vi "Periodic Tasks.vi"(8 "error in":errorcluster) -> ()   [LabVIEW 2016]
doc: "This VI runs in parallel to other tasks. It can contain as many user-defined periodic loops as you need. These can carry out PID or other sorts of timed response."
uses:
  Control 1.ctl
  <vilib>/Platform/TimedLoop/XDataNode/timing_clust.ctl
  <vilib>/Platform/TimedLoop/XDataNode/nitl_modes.ctl
  <vilib>/Platform/TimedLoop/XDataNode/wakeup.ctl
  <userlib>/836-Library/Drive/Drive_Code_V2/Drive_Code_Support/SensorTypedefs/Sensor_Cluster.ctl
  <userlib>/836-Library/Drive/Drive_Code_V2/Drive_Code_Support/SensorTypedefs/Camera_Cluster.ctl
  <vilib>/Rock Robotics/WPI/RobotDrive/WPI_RobotDriveDevRef.ctl
  <vilib>/Rock Robotics/WPI/MotorControl/WPI_MotorControlDeviceRef.ctl
  <vilib>/Rock Robotics/WPI/MotorControl/WPI_MotorControlType.ctl
  <vilib>/Rock Robotics/SystemInterfaces/DIO/FPGA_DIOPWMChannel.ctl
  <vilib>/Rock Robotics/WPI/PWM/WPI_PWMDeadband.ctl
  <userlib>/836-Library/Drive/Drive_Code_V2/Drive_Code_Support/DriveTrains/Drive_Trains.ctl
  <userlib>/836-Library/Drive/Drive_Code_V2/Drive_Code_Support/Command_Sends/Drive_Code_Command_Type.ctl
  <userlib>/836-Library/Drive/Drive_Code_V2/Drive_Code_Support/Command_Sends/Drive_Code_Command_List.ctl
  <userlib>/836-Library/Drive/Drive_Code_V2/Drive_Code_Support/PidClusters/PidInversions.ctl
  <userlib>/836-Library/Drive/Drive_Code_V2/Drive_Code_Support/PidClusters/DrivePidInputs.ctl
  <userlib>/836-Library/Drive/Drive_Code_V2/Drive_Code_Support/PidClusters/PidInputs.ctl
  <userlib>/836-Library/Drive/Drive_Code_V2/Drive_Code_Support/Command_Sends/Command_Tolerances.ctl
  <userlib>/836-Library/Drive/Drive_Code_V2/Drive_Code_Support/Command_Sends/Command_Tolerance_Info.ctl
  <vilib>/Rock Robotics/WPI/Utilities/WPI_GetSetVariantRefNum.vi
  <userlib>/836-Library/Drive/Drive_Code_V2/Drive_Code_Support/Command_Sends/Drive_Cmd_Cheesey_Drive.vi
  <vilib>/platform/TimedLoop/XDataNode/XDataNode.xnode
  <vilib>/Platform/TimedLoop/XDataNode/XDNodeRunTimeDep.lvlib
panel:
  in  "Tab Control":T1(tab)=enum."Motor_9"
  in  "Press and Hold? 4":T2=TRUE
  in  "Reverse Direction? 4":bool
  in  "Power 4":dbl(knob) scale=0.0..1.0
  in  "Press and Hold? 5":T2=TRUE
  in  "Reverse Direction? 5":bool
  in  "Power 5":dbl(knob) scale=0.0..1.0
  in  "Press and Hold? 6":T2=TRUE
  in  "Reverse Direction? 6":bool
  in  "Power 6":dbl(knob) scale=0.0..1.0
  in  "Press and Hold? 7":T2=TRUE
  in  "Reverse Direction? 7":bool
  in  "Power 7":dbl(knob) scale=0.0..1.0
  in  "Rev Press and Hold? 8":T2=TRUE
  in  "Rev Power 8":dbl(knob) scale=0.0..1.0
  in  "Fwd Press and Hold? 8":T2=TRUE
  in  "Reverse Direction? 8":bool
  in  "Fwd Power 8":dbl(knob) scale=0.0..1.0
  in  "Rev Press and Hold? 9":T2=TRUE
  in  "Rev Power 9":dbl(knob) scale=0.0..1.0
  in  "Fwd Press and Hold? 9":T2=TRUE
  in  "Reverse Direction? 9":bool
  in  "Fwd Power 9":dbl(knob) scale=0.0..1.0
  # "PWM: 4\nButton: X"
  # "PWM: 5\nButton: A"
  # "PWM: 6\nButton: B"
  # "PWM: 7\nButton: Y"
  # "PWM: 8\nFwd Button: RB\nRev Button: LB"
  # "PWM: 9\nFwd Button: RT\nRev Button: LT"
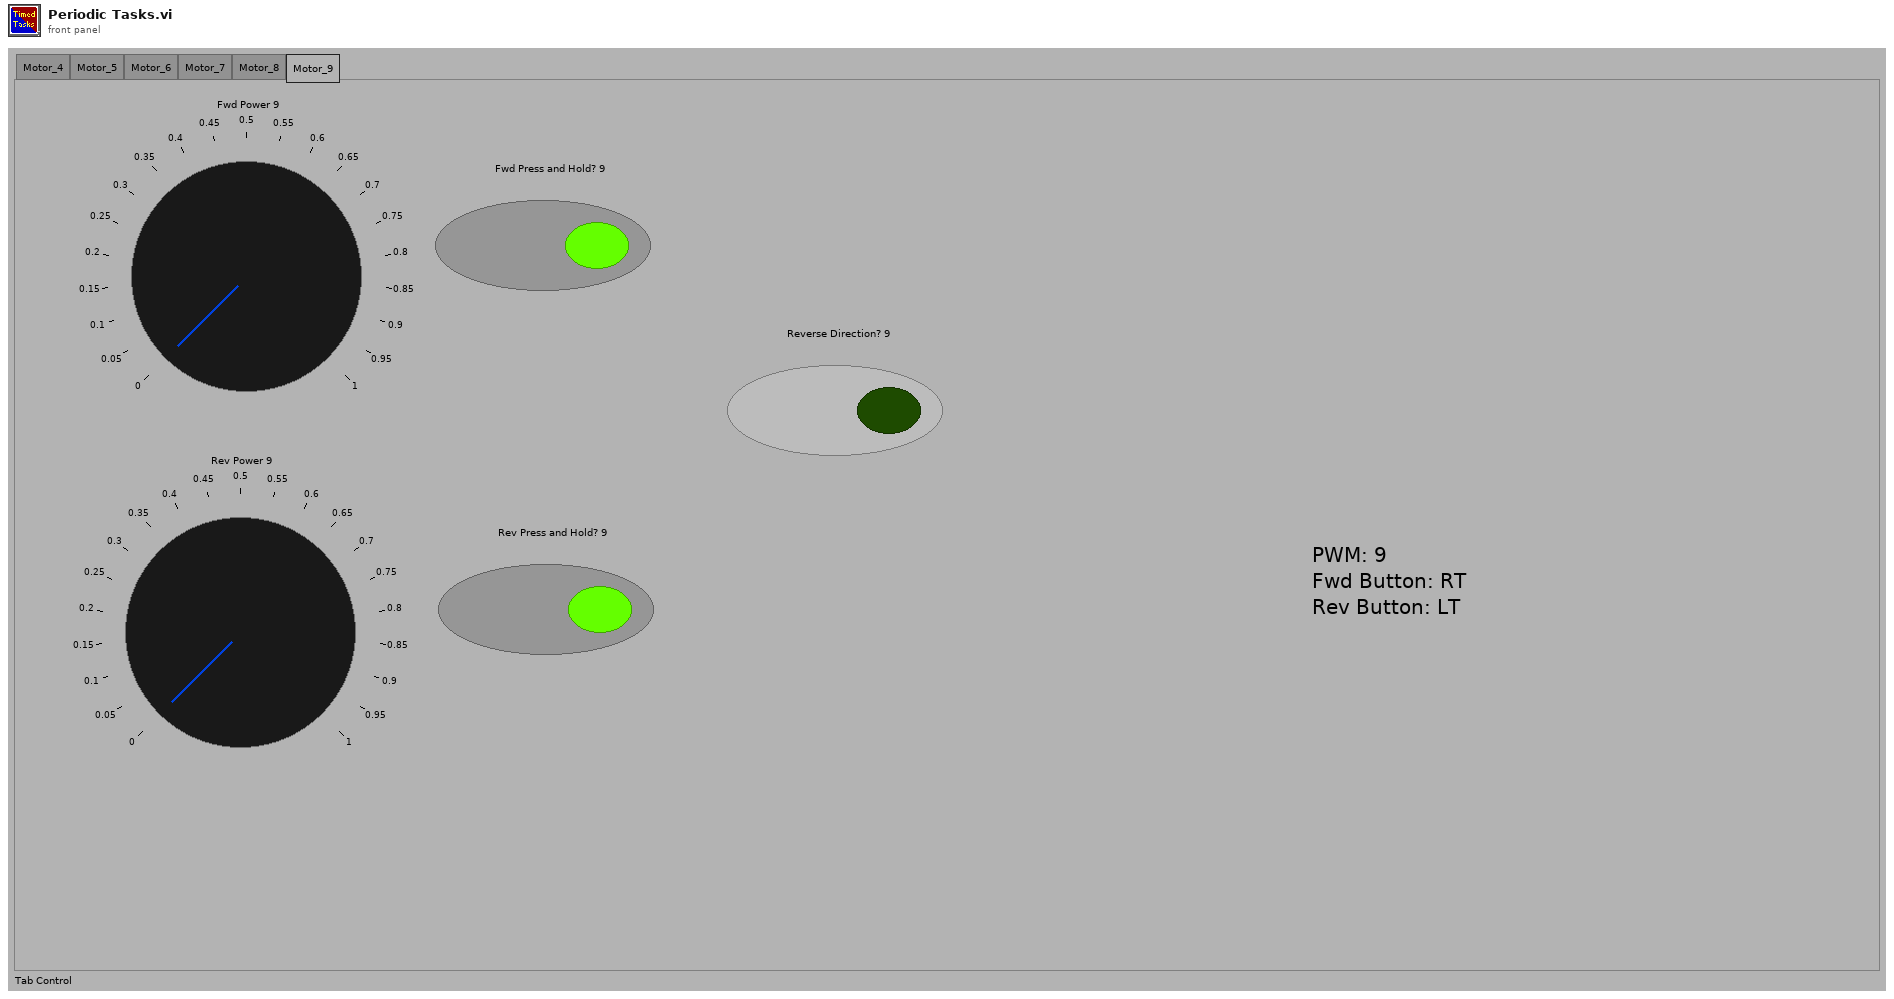
[diagram p1: front panel]
types:
  T1 = enum32{"Motor_4", "Motor_5", "Motor_6", "Motor_7", "Motor_8", "Motor_9"}
  T2 = typedef "Control 1.ctl" = bool
  T3 = typedef "XDNodeRunTimeDep.lvlib/timing_clust.ctl" = cluster{"Expected End [f-1]":u64, "Actual End [f-1]":u64, "Finished Late? [f-1]":bool, "Expected End [i-1]":u64, "Actual End [i-1]":u64, "Finished Late? [i-1]":bool, "Expected Start [i]":u64, "Actual Start [i]":u64, "Expected Start [f]":u64, "Actual Start [f]":u64, "Source Name":string, "Structure Name":string, "Period":i64, "Deadline":i64, "Offset":i64, "Start":i64, "Priority":i32, "Timeout":i32, "Mode":T4, "Wakeup Reason":T5, "Error":errorcluster, "Source Type":string, "Secondary Source Type":string, "Global End Time":u64, "Global Start Time":u64, "Frame Duration":u64, "Iteration Duration":u64, "Assigned CPU":i32, "I/O Scan Engine Mode":u32}
  T4 = typedef "XDNodeRunTimeDep.lvlib/nitl_modes.ctl" = enum32{"No Change", "Process missed periods, maintain original phase", "Discard missed periods, maintain original phase", "Process missed periods, ignore original phase", "Discard missed periods, ignore original phase"}
  T5 = typedef "XDNodeRunTimeDep.lvlib/wakeup.ctl" = enum32{"Normal", "Aborted", "Asynchronous wakeup", "Timing source error", "Timed loop error", "Timeout"}
  T6 = cluster{"Rev Power":dbl, "Rev Press and Hold?":T2}
  T7 = cluster{"Fwd Power":dbl, "Fwd Press and Hold?":T2}
  T8 = typedef "WPI_JoystickDevRef.ctl" = cluster{"Device":T9}
  T9 = typedef "WPI_JoystickDeviceEnum.ctl" = enum16{"USB 0", "USB 1", "USB 2", "USB 3", "USB 4", "USB 5"}
  T10 = typedef "Sensor_Cluster.ctl" = cluster{"Gyro Data":cluster{"Gyro RT FIFO":refnum<k33>, "Gyro Current":dbl, "Gyro Hold":dbl}, "Encoder Data":cluster{"Encoder RT FIFO":refnum<k33>, "Encoder Current":dbl, "Encoder Hold":dbl}, "Camera Data":cluster{"Camera RT FIFO":refnum<k33>, "Camera Current":T11}}
  T11 = typedef "Camera_Cluster.ctl" = cluster{" Angle":dbl, "Valid":bool}
  T12 = typedef "WPI_RobotDriveDevRef.ctl" = cluster{"DevStatus":errorcluster, "Motors[]":T13[], "Square Inputs":bool, "Max Output":dbl}
  T13 = typedef "WPI_MotorControlDeviceRef.ctl" = cluster{"DeviceStatus":errorcluster, "Type":T14, "PWM":cluster{"PWM Channel":T15, "DeadBand":T16}, "CAN":cluster{"Device Number":u8, "SetOutput VI Ref":variant, "GetOutput VI Ref":variant, "Enable VI Ref":variant, "Disable VI Ref":variant, "Data":variant}, "Invert":bool}
  T14 = typedef "WPI_MotorControlType.ctl" = enum16{"PWM", "CAN"}
  T15 = typedef "FPGA_DIOPWMChannel.ctl" = enum8{"PWM 0", "PWM 1", "PWM 2", "PWM 3", "PWM 4", "PWM 5", "PWM 6", "PWM 7", "PWM 8", "PWM 9", "PWM MXP 0", "PWM MXP 1", "PWM MXP 2", "PWM MXP 3", "PWM MXP 4", "PWM MXP 5", "PWM MXP 6", "PWM MXP 7", "PWM MXP 8", "PWM MXP 9", "Invalid"}
  T16 = typedef "WPI_PWMDeadband.ctl" = cluster{"Name":string, "maxPositivePwm":i32, "minPositivePwm":i32, "centerPwm":i32, "maxNegativePwm":i32, "minNegativePwm":i32, "angularRange":u16}
  T17 = typedef "Drive_Trains.ctl" = enum16{"Tank Drive 2 Motor", "Tank Drive 4 Motor", "Mecanum Drive", "Kiwi Drive"}
  T18 = typedef "PidInversions.ctl" = cluster{"Distance PID Inverted?":bool, "Yaw PID Inverted?":bool}
  T19 = cluster{"Cluster":T10, "RobotDriveDevRef":T12, "Drive Train":T17, "Valid Commands":bool[], "Drive Comand Notifier":refnum<notifier>, "Command Finished?":refnum<k4>, "Command Canceled":refnum<k4>, "PID Inversions":T18, "PID Inputs Notifier":refnum<notifier>, "Cmd Tol Notifier":refnum<notifier>}
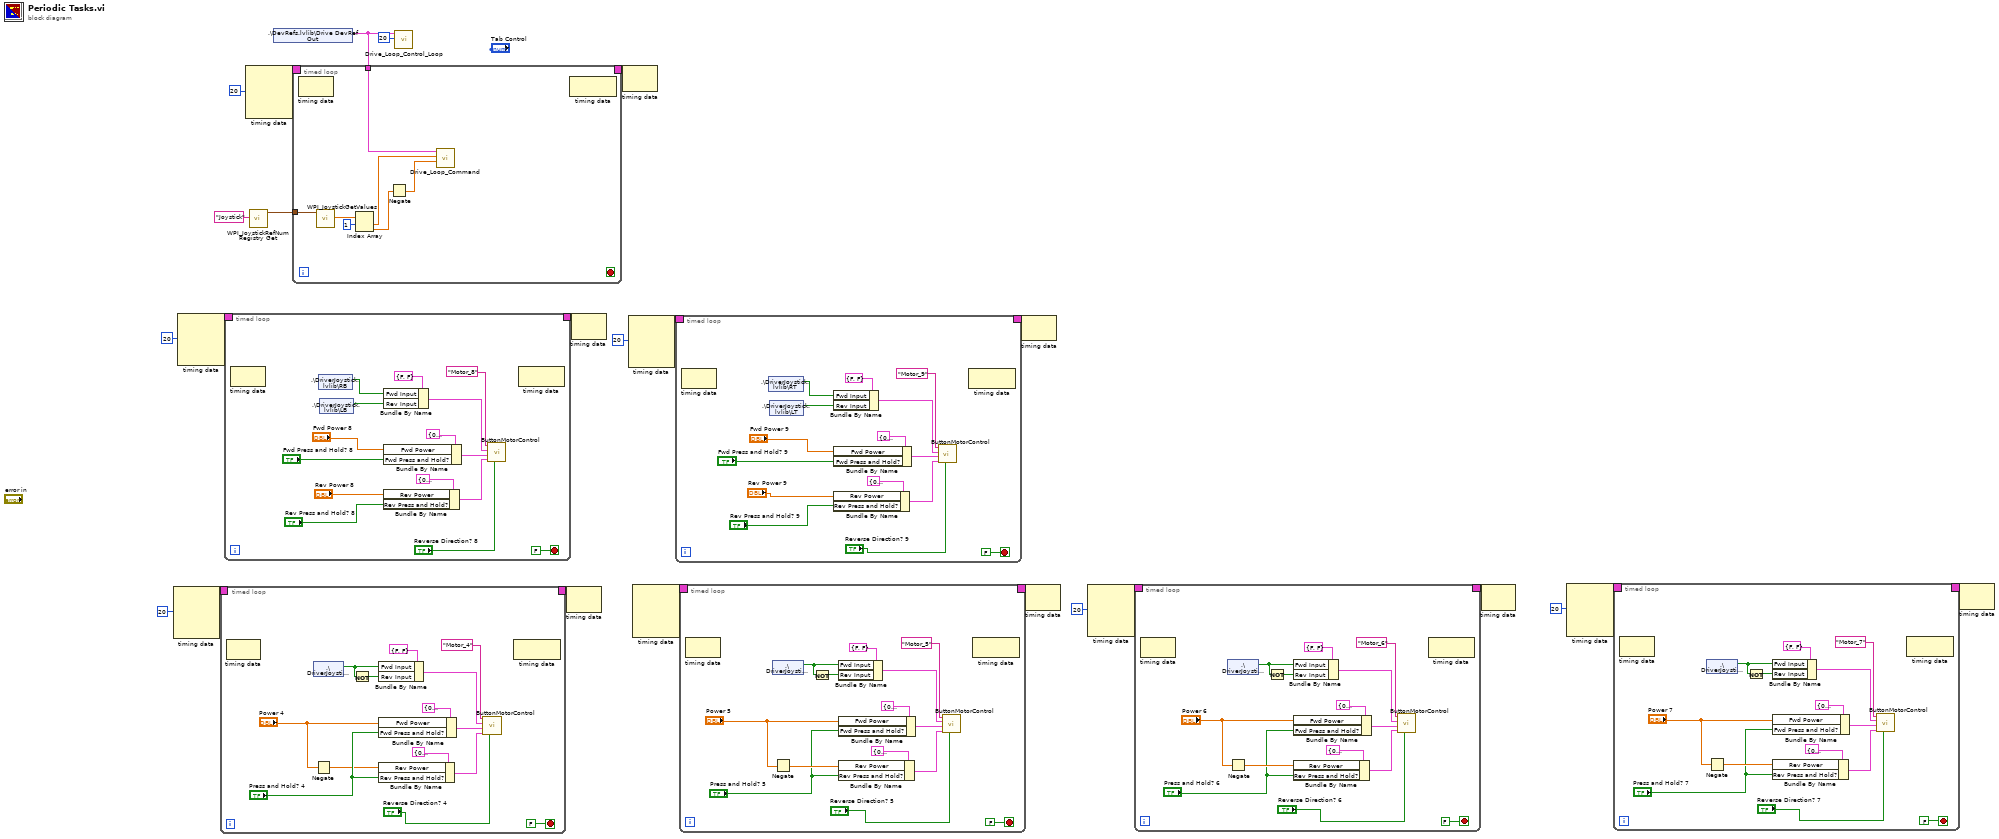
[diagram p0: block diagram]
diagram:
  n1 = node-c288(i64 20 ("Period")) -> (w12:T3)  [unwired: 3 in]
  n2 = node-c288(i64 20 ("Period")) -> (w17:T3)  [unwired: 3 in]
  n3 = timed-loop {
    timing: w12 -> [_]
    timing-out: [_] -> w11
    stop <- FALSE stop-if-true
    n4 = node-c288() -> ()  [unwired: 1 in, 1 out]
    n5 = shared-variable ".\\DriverJoystick.lvlib\\X"() -> (w30:bool)  [unwired: 1 in, 1 out]
    n6 = Negate(x="Power 4") -> (-x=w27:dbl)
    n7 = Not(x=w30) -> (.not. x?=w29:bool)
    n8 = Bundle By Name(cluster=cluster{"Fwd Input":bool, "Rev Input":bool} {"Fwd Input"=FALSE, "Rev Input"=FALSE} ("Input"), "Fwd Input"=w30, "Rev Input"=w29) -> (w36:cluster{"Fwd Input":bool, "Rev Input":bool})
    n9 = Bundle By Name(cluster=T7 {"Fwd Power"=0.0, "Fwd Press and Hold?"=TRUE} ("Fwd Config"), "Fwd Power"="Power 4", "Fwd Press and Hold?"="Press and Hold? 4") -> (w34:T7)
    n10 = Bundle By Name(cluster=T6 {"Rev Power"=0.0, "Rev Press and Hold?"=TRUE} ("Rev Config"), "Rev Power"=w27, "Rev Press and Hold?"="Press and Hold? 4") -> (w32:T6)
    n11 = call "ButtonMotorControl.vi"("Reverse Direction?"="Reverse Direction? 4", "Rev Config"=w32, "Fwd Config"=w34, "Input"=w36, "Motor Name"="Motor_4") -> ()  [unwired: 7 in]
    n12 = node-c288() -> ()  [unwired: 1 in, 1 out]
  }
  n13 = timed-loop {
    timing: w17 -> [_]
    timing-out: [_] -> w16
    stop <- FALSE stop-if-true
    n14 = node-c288() -> ()  [unwired: 1 in, 1 out]
    n15 = shared-variable ".\\DriverJoystick.lvlib\\RB"() -> (w53:bool)  [unwired: 1 in, 1 out]
    n16 = shared-variable ".\\DriverJoystick.lvlib\\LB"() -> (w52:bool)  [unwired: 1 in, 1 out]
    n17 = Bundle By Name(cluster=cluster{"Fwd Input":bool, "Rev Input":bool} {"Fwd Input"=FALSE, "Rev Input"=FALSE} ("Input"), "Fwd Input"=w53, "Rev Input"=w52) -> (w51:cluster{"Fwd Input":bool, "Rev Input":bool})
    n18 = Bundle By Name(cluster=T7 {"Fwd Power"=0.0, "Fwd Press and Hold?"=TRUE} ("Fwd Config"), "Fwd Power"="Fwd Power 8", "Fwd Press and Hold?"="Fwd Press and Hold? 8") -> (w46:T7)
    n19 = Bundle By Name(cluster=T6 {"Rev Power"=0.0, "Rev Press and Hold?"=TRUE} ("Rev Config"), "Rev Power"="Rev Power 8", "Rev Press and Hold?"="Rev Press and Hold? 8") -> (w42:T6)
    n20 = call "ButtonMotorControl.vi"("Reverse Direction?"="Reverse Direction? 8", "Rev Config"=w42, "Fwd Config"=w46, "Input"=w51, "Motor Name"="Motor_8") -> ()  [unwired: 7 in]
    n21 = node-c288() -> ()  [unwired: 1 in, 1 out]
  }
  n22 = node-c288(i64 20 ("Period")) -> (w24:T3)  [unwired: 3 in]
  n23 = call <vilib>:"WPI_JoystickRefNum Registry Get.vi"("refnum name"="Joystick") -> ("JoystickDevRef"=w19:T8)  [unwired: 9 in, 1 out]
  n24 = shared-variable ".\\DevRefs.lvlib\\Drive DevRef Out"() -> (w22:T19)  [unwired: 1 in, 1 out]
  n25 = timed-loop {
    timing: w24 -> [_]
    timing-out: [_] -> w23
    tunnel: w22 -> [w64]
    tunnel: w19 -> [w63]
    stop <- _ stop-if-true
    n26 = node-c288() -> ()  [unwired: 1 in, 1 out]
    n27 = call <vilib>:"WPI_JoystickGetValues.vi"("JoystickDevRef"=w63) -> ("Axes"=w62:dbl[])  [unwired: 6 in, 4 out]
    n28 = Index Array(array=w62, index #1=1 ("index")) -> (element #1=w60:dbl, element #2=w59:dbl)  [unwired: 1 in]
    n29 = Negate(x=w59) -> (-x=w58:dbl)
    n30 = call-poly <userlib>:"Drive_Loop_Command.vi"("Wheel"=w58, "Throttle"=w60, "Drive Loop Cluster"=w64) -> ()  [unwired: 8 in, 1 out]
    n31 = node-c288() -> ()  [unwired: 1 in, 1 out]
  }
  n32 = call <userlib>:"Drive_Loop_Control_Loop.vi"("Init Period"=i64 20, "Drive DevRef In"=w22) -> ()  [unwired: 10 in]
  n33 = node-c288(w11) -> ()  [unwired: 1 out]
  n34 = node-c288(w16) -> ()  [unwired: 1 out]
  n35 = node-c288(w23) -> ()  [unwired: 1 out]
  n36 = node-c288(i64 20 ("Period")) -> (w14:T3)  [unwired: 3 in]
  n37 = node-c288() -> (w8:T3)  [unwired: 4 in]
  n38 = timed-loop {
    timing: w14 -> [_]
    timing-out: [_] -> w13
    stop <- FALSE stop-if-true
    n39 = node-c288() -> ()  [unwired: 1 in, 1 out]
    n40 = shared-variable ".\\DriverJoystick.lvlib\\RT"() -> (w79:bool)  [unwired: 1 in, 1 out]
    n41 = shared-variable ".\\DriverJoystick.lvlib\\LT"() -> (w78:bool)  [unwired: 1 in, 1 out]
    n42 = Bundle By Name(cluster=cluster{"Fwd Input":bool, "Rev Input":bool} {"Fwd Input"=FALSE, "Rev Input"=FALSE} ("Input"), "Fwd Input"=w79, "Rev Input"=w78) -> (w77:cluster{"Fwd Input":bool, "Rev Input":bool})
    n43 = Bundle By Name(cluster=T7 {"Fwd Power"=0.0, "Fwd Press and Hold?"=TRUE} ("Fwd Config"), "Fwd Power"="Fwd Power 9", "Fwd Press and Hold?"="Fwd Press and Hold? 9") -> (w75:T7)
    n44 = Bundle By Name(cluster=T6 {"Rev Power"=0.0, "Rev Press and Hold?"=TRUE} ("Rev Config"), "Rev Power"="Rev Power 9", "Rev Press and Hold?"="Rev Press and Hold? 9") -> (w73:T6)
    n45 = call "ButtonMotorControl.vi"("Reverse Direction?"="Reverse Direction? 9", "Rev Config"=w73, "Fwd Config"=w75, "Input"=w77, "Motor Name"="Motor_9") -> ()  [unwired: 7 in]
    n46 = node-c288() -> ()  [unwired: 1 in, 1 out]
  }
  n47 = timed-loop {
    timing: w8 -> [_]
    timing-out: [_] -> w7
    stop <- FALSE stop-if-true
    n48 = node-c288() -> ()  [unwired: 1 in, 1 out]
    n49 = shared-variable ".\\DriverJoystick.lvlib\\A"() -> (w89:bool)  [unwired: 1 in, 1 out]
    n50 = Negate(x="Power 5") -> (-x=w87:dbl)
    n51 = Not(x=w89) -> (.not. x?=w88:bool)
    n52 = Bundle By Name(cluster=cluster{"Fwd Input":bool, "Rev Input":bool} {"Fwd Input"=FALSE, "Rev Input"=FALSE} ("Input"), "Fwd Input"=w89, "Rev Input"=w88) -> (w95:cluster{"Fwd Input":bool, "Rev Input":bool})
    n53 = Bundle By Name(cluster=T7 {"Fwd Power"=0.0, "Fwd Press and Hold?"=TRUE} ("Fwd Config"), "Fwd Power"="Power 5", "Fwd Press and Hold?"="Press and Hold? 5") -> (w93:T7)
    n54 = Bundle By Name(cluster=T6 {"Rev Power"=0.0, "Rev Press and Hold?"=TRUE} ("Rev Config"), "Rev Power"=w87, "Rev Press and Hold?"="Press and Hold? 5") -> (w91:T6)
    n55 = call "ButtonMotorControl.vi"("Reverse Direction?"="Reverse Direction? 5", "Rev Config"=w91, "Fwd Config"=w93, "Input"=w95, "Motor Name"="Motor_5") -> ()  [unwired: 7 in]
    n56 = node-c288() -> ()  [unwired: 1 in, 1 out]
  }
  n57 = node-c288(w13) -> ()  [unwired: 1 out]
  n58 = node-c288(w7) -> ()  [unwired: 1 out]
  n59 = node-c288(i64 20 ("Period")) -> (w6:T3)  [unwired: 3 in]
  n60 = timed-loop {
    timing: w6 -> [_]
    timing-out: [_] -> w5
    stop <- FALSE stop-if-true
    n61 = node-c288() -> ()  [unwired: 1 in, 1 out]
    n62 = shared-variable ".\\DriverJoystick.lvlib\\B"() -> (w105:bool)  [unwired: 1 in, 1 out]
    n63 = Negate(x="Power 6") -> (-x=w103:dbl)
    n64 = Not(x=w105) -> (.not. x?=w104:bool)
    n65 = Bundle By Name(cluster=cluster{"Fwd Input":bool, "Rev Input":bool} {"Fwd Input"=FALSE, "Rev Input"=FALSE} ("Input"), "Fwd Input"=w105, "Rev Input"=w104) -> (w111:cluster{"Fwd Input":bool, "Rev Input":bool})
    n66 = Bundle By Name(cluster=T7 {"Fwd Power"=0.0, "Fwd Press and Hold?"=TRUE} ("Fwd Config"), "Fwd Power"="Power 6", "Fwd Press and Hold?"="Press and Hold? 6") -> (w109:T7)
    n67 = Bundle By Name(cluster=T6 {"Rev Power"=0.0, "Rev Press and Hold?"=TRUE} ("Rev Config"), "Rev Power"=w103, "Rev Press and Hold?"="Press and Hold? 6") -> (w107:T6)
    n68 = call "ButtonMotorControl.vi"("Reverse Direction?"="Reverse Direction? 6", "Rev Config"=w107, "Fwd Config"=w109, "Input"=w111, "Motor Name"="Motor_6") -> ()  [unwired: 7 in]
    n69 = node-c288() -> ()  [unwired: 1 in, 1 out]
  }
  n70 = node-c288(w5) -> ()  [unwired: 1 out]
  n71 = node-c288(i64 20 ("Period")) -> (w3:T3)  [unwired: 3 in]
  n72 = timed-loop {
    timing: w3 -> [_]
    timing-out: [_] -> w2
    stop <- FALSE stop-if-true
    n73 = node-c288() -> ()  [unwired: 1 in, 1 out]
    n74 = shared-variable ".\\DriverJoystick.lvlib\\Y"() -> (w121:bool)  [unwired: 1 in, 1 out]
    n75 = Negate(x="Power 7") -> (-x=w119:dbl)
    n76 = Not(x=w121) -> (.not. x?=w120:bool)
    n77 = Bundle By Name(cluster=cluster{"Fwd Input":bool, "Rev Input":bool} {"Fwd Input"=FALSE, "Rev Input"=FALSE} ("Input"), "Fwd Input"=w121, "Rev Input"=w120) -> (w127:cluster{"Fwd Input":bool, "Rev Input":bool})
    n78 = Bundle By Name(cluster=T7 {"Fwd Power"=0.0, "Fwd Press and Hold?"=TRUE} ("Fwd Config"), "Fwd Power"="Power 7", "Fwd Press and Hold?"="Press and Hold? 7") -> (w125:T7)
    n79 = Bundle By Name(cluster=T6 {"Rev Power"=0.0, "Rev Press and Hold?"=TRUE} ("Rev Config"), "Rev Power"=w119, "Rev Press and Hold?"="Press and Hold? 7") -> (w123:T6)
    n80 = call "ButtonMotorControl.vi"("Reverse Direction?"="Reverse Direction? 7", "Rev Config"=w123, "Fwd Config"=w125, "Input"=w127, "Motor Name"="Motor_7") -> ()  [unwired: 7 in]
    n81 = node-c288() -> ()  [unwired: 1 in, 1 out]
  }
  n82 = node-c288(w2) -> ()  [unwired: 1 out]
